vi "KaKbParameter.vi"(6 "Impedance Z (10m)":dbl=0.01 min=0.01 max=100000000.0 format="%^.2e", 7 "Frequency (20)":dbl=20.0 min=20.0 max=1000000.0 format="%.2f", 8 "error in (no error)":errorcluster, 9 "Integ Time (0: Short)":enum16{"SHORT", "MED/LONG"}(ring), 10 "Voltage Level (1.0)":dbl=1.0 min=0.005 max=20.0 format="%.3f", 11 "VISA resource name":refnum<visa-resource-name>) -> (0 "error out":errorcluster, 1 "Ka":dbl format="%^.2e", 2 "Kb":dbl format="%^.2e", 3 "VISA resource name out":refnum<visa-resource-name>)   [LabVIEW 2015, in "Agilent 428X Series.lvlib"]
doc: "This VI computes the value of impedance Proportional Factors Ka and Kb, Returned result can be verified by checking table9-1.\n\n Freq. Ka \n---------------------------------------------------------------------------------------------------------\n f<100Hz (1*10E-3)/Z*(1+200/Vs)*(1+sqrt(100/fm))\nMed/Long 100<f<100k (1*10E-3)/Z*(1+200/Vs) \n 100k<f<300k (1*10E-3)/Z*(2+200/Vs)\n 300k<f<1M (1*10E-3)/Z*(3+200/Vs+Vs^2/1E8)\n---------------------------------------------------------------------------------------------------------\n f<100Hz (2.5*1E-3)/Z*(1+400/Vs)*(1+sqrt(100/fm))\nSHORT 100<f<100k (2.5*10E-3)/Z*(1+400/Vs) \n 100k<f<300k (2.5*10E-3)/Z*(2+400/Vs)\n 300k<f<1M (2.5*10E-3)/Z*(3+400/Vs+Vs^2/1E8)\n---------------------------------------------------------------------------------------------------------\n\n Freq. Kb \n---------------------------------------------------------------------------------------------------------\n f<100Hz (1*1E-9)*Z*(1+70/Vs)*(1+sqrt(100/fm))\nMed/Long 100<f<100k (1*1E-9)*Z*(1+70/Vs) \n 100k<f<300k (3*1E-9)*Z*(1+70/Vs)\n 300k<f<1M (1E-8)*Z*(1+70/Vs)\n---------------------------------------------------------------------------------------------------------\n f<100Hz (2*1E-9)*Z*(1+100/Vs)*(1+sqrt(100/fm))\nSHORT 100<f<100k (2*1E-9)*Z*(1+100/Vs) \n 100k<f<300k (6*1E-9)*Z*(2+100/Vs)\n 300k<f<1M (20*1E-9)*Z*(1+100/Vs)\n---------------------------------------------------------------------------------------------------------\n\nDisclaimer: All accuracy calculation VI's are not part of the original \n driver. They are provided for supplementry purpose only.\n If user desires very high accuracy data, please do or \n check the calculation seperately."
uses:
  Agilent 428X Series.lvlib
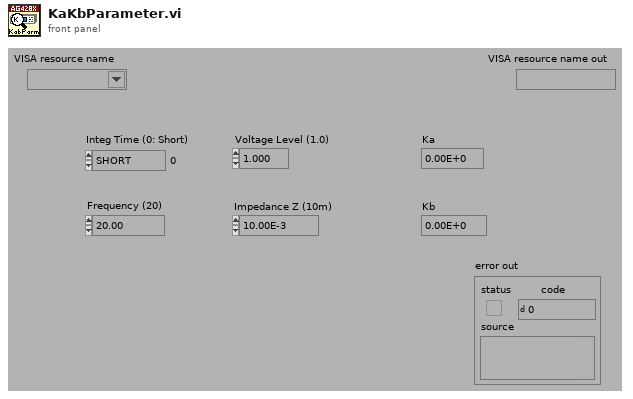
[diagram p1: front panel]
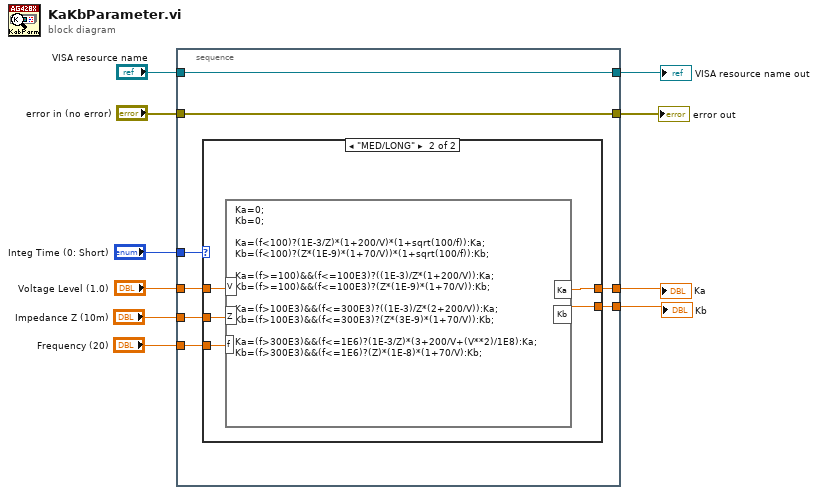
[diagram p0: block diagram]
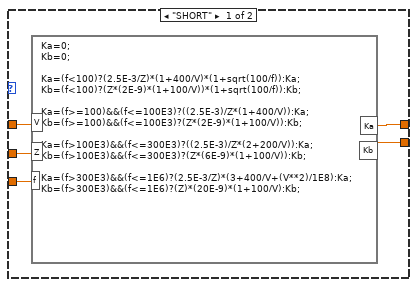
[diagram p2: hidden frame]
diagram:
  n1 = stacked-sequence {
    tunnel: "Integ Time (0: Short)" -> [w18]
    tunnel: "Voltage Level (1.0)" -> [w17]
    tunnel: "Impedance Z (10m)" -> [w16]
    tunnel: "Frequency (20)" -> [w15]
    tunnel: "error in (no error)" -> [w14]
    tunnel: [w14] -> w5
    tunnel: "VISA resource name" -> [w13]
    tunnel: [w13] -> w3
    tunnel: [w12] -> w2
    tunnel: [w11] -> w1
    frame #0 {
      n2 = case shown="\"MED/LONG\"" w18 {
        tunnel: w17 -> [w23 w28]
        tunnel: w16 -> [w22 w27]
        tunnel: w15 -> [w21 w26]
        tunnel: [w20 w25] -> w12
        tunnel: [w19 w24] -> w11
        frame "SHORT" {
          n3 = formula code="Ka=0;\nKb=0;\n\nKa=(f<100)?(2.5E-3/Z)*(1+400/V)*(1+sqrt(100/f)):Ka;\nKb=(f<100)?(Z*(2E-9)*(1+100/V))*(1+sqrt(100/f)):Kb;\n\nKa=(f>=100)&&(f<=100E3)?((2.5E-3)/Z*(1+400/V)):Ka;\nKb=(f>=100)&&(f<=100E3)?(Z*(2E-9)*(1+100/V)):Kb;\n\nKa=(f>100E3)&&(f<=300E3)?((2.5E-3)/Z*(2+200/V)):Ka;\nKb=(f>100E3)&&(f<=300E3)?(Z*(6E-9)*(1+100/V)):Kb;\n\nKa=(f>300E3)&&(f<=1E6)?(2.5E-3/Z)*(3+400/V+(V**2)/1E8):Ka;\nKb=(f>300E3)&&(f<=1E6)?(Z)*(20E-9)*(1+100/V):Kb;"("V"=w23, "Z"=w22, "f"=w21) -> ("Ka"=w20:dbl, "Kb"=w19:dbl)
        }
        frame "MED/LONG" {
          n4 = formula code="Ka=0;\nKb=0;\n\nKa=(f<100)?(1E-3/Z)*(1+200/V)*(1+sqrt(100/f)):Ka;\nKb=(f<100)?(Z*(1E-9)*(1+70/V))*(1+sqrt(100/f)):Kb;\n\nKa=(f>=100)&&(f<=100E3)?((1E-3)/Z*(1+200/V)):Ka;\nKb=(f>=100)&&(f<=100E3)?(Z*(1E-9)*(1+70/V)):Kb;\n\nKa=(f>100E3)&&(f<=300E3)?((1E-3)/Z*(2+200/V)):Ka;\nKb=(f>100E3)&&(f<=300E3)?(Z*(3E-9)*(1+70/V)):Kb;\n\nKa=(f>300E3)&&(f<=1E6)?(1E-3/Z)*(3+200/V+(V**2)/1E8):Ka;\nKb=(f>300E3)&&(f<=1E6)?(Z)*(1E-8)*(1+70/V):Kb;"("V"=w28, "Z"=w27, "f"=w26) -> ("Ka"=w25:dbl, "Kb"=w24:dbl)
        }
      }
    }
  }
  "VISA resource name out" <- w3
  "error out" <- w5
  "Ka" <- w2
  "Kb" <- w1
